vi "Simple Digital Input.vi"() -> ()   [LabVIEW 2015]
doc: "This example shows how to read values from a digital channel.\n\nIt will display the digital value as Low (LED off) or High (LED on).\n\nThis example expects a USB cable connected from your development PC to the Type B USB Jack (next to the power input) on the roboRIO."
uses:
  <vilib>/Rock Robotics/SystemInterfaces/DIO/FPGA_DIOChannel.ctl
panel:
  out "Digital Input Value":bool
  in  "DIO Channel":T1=enum."DIO 6"
  in  "stop":bool
  # "Set this input before running."
  # "TTL Signal"
  # "This shows wiring for a TTL signal.  To read a switch, wire one side of the switch to DIO-6 S and the other side to DIO-6 ground.  The LED will be On when the switch is open and Off when the switch is closed."
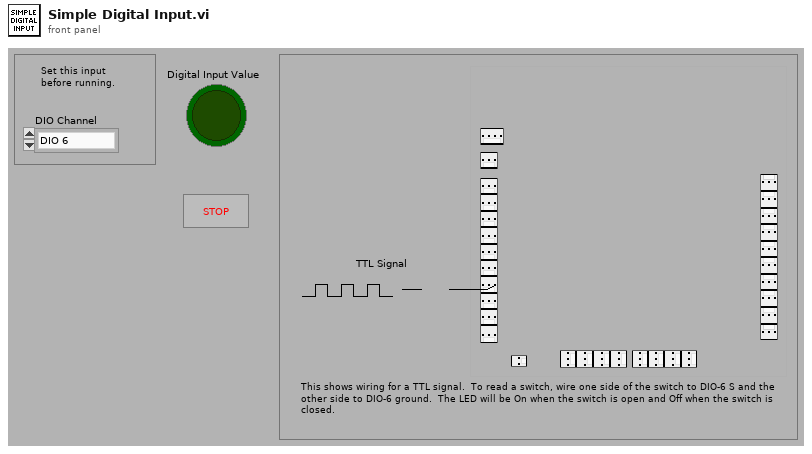
[diagram p1: front panel]
types:
  T1 = typedef "FPGA_DIOChannel.ctl" = enum8{"DIO 0", "DIO 1", "DIO 2", "DIO 3", "DIO 4", "DIO 5", "DIO 6", "DIO 7", "DIO 8", "DIO 9", "DIO MXP 0", "DIO MXP 1", "DIO MXP 2", "DIO MXP 3", "DIO MXP 4", "DIO MXP 5", "DIO MXP 6", "DIO MXP 7", "DIO MXP 8", "DIO MXP 9", "DIO MXP 10", "DIO MXP 11", "DIO MXP 12", "DIO MXP 13", "DIO MXP 14", "DIO MXP 15", "Invalid"}
  T2 = typedef "WPI_DigitalInputDevRef.ctl" = cluster{"DevStatus":errorcluster, "DIO Channel":T1}
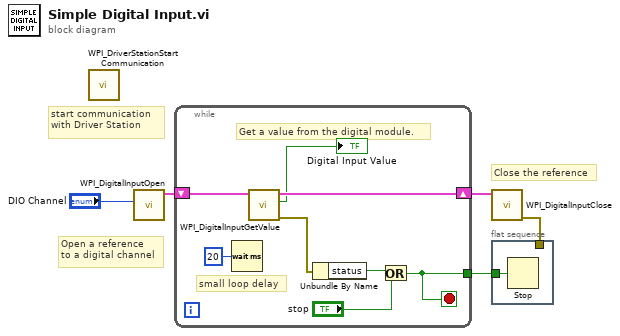
[diagram p0: block diagram]
diagram:
  # "start communication with Driver Station"
  # "Close the reference"
  # "Open a reference\nto a digital channel"
  n1 = call <vilib>:"WPI_DriverStationStart Communication.vi"() -> ()  [unwired: 2 in, 10 out]
  n2 = call <vilib>:"WPI_DigitalInputOpen.vi"("DIO Channel"="DIO Channel") -> ("DigitalInputDevRef"=w4:T2)  [unwired: 1 in, 9 out]
  n3 = while {
    shift-right: [w12] -> w3
    shift-left: w4 -> [w13]
    tunnel: [w9] -> w2
    stop <- w9 stop-if-true
    # "small loop delay"
    # "Get a value from the digital module."
    n4 = Wait (ms)(milliseconds to wait=u32 20) -> ()  [unwired: 1 out]
    n5 = call <vilib>:"WPI_DigitalInputGetValue.vi"("DigitalInputDevRef"=w13) -> ("error out"=w8:errorcluster, "Value"=→"Digital Input Value":bool, "DigitalInputDevRef"=w12:T2)  [unwired: 1 in, 7 out]
    n6 = Unbundle By Name(w8) -> ("status"=w10:bool)
    n7 = Or(x=w10, y="stop") -> (x .or. y?=w9:bool)
  }
  n8 = call <vilib>:"WPI_DigitalInputClose.vi"("DigitalInputDevRef"=w3) -> ("error out"=w1:errorcluster)  [unwired: 1 in, 9 out]
  n9 = flat-sequence {
    tunnel: w2 -> [w14]
    tunnel: w1 -> [_]
    frame #0 {
      n10 = Stop(stop? (T)=w14) -> ()
    }
  }
